vi "Secondary Master.vi"() -> ()   [LabVIEW 2021]
doc: "Secondary Modbus master that reads from a holding register periodically to ensure the primary master is functioning properly. If the holding register fails to update for a period of time, the secondary master assumes all the duties of the primary."
uses:
  Modbus_v121c/API/Modbus API.lvclass/Modbus API.ctl
  Modbus_v121c/API/Read Network Protocol.vi
  Modbus_v121c/API/Master/Modbus Master.lvclass
  D:/my_projects/projects/Algorithms/Labview/21/Modbus_v121c/API/Modbus API.lvclass
  Modbus_v121c/API/Wrapper/Create TCP Master.vi
  Stop Global.vi
  Modbus_v121c/Network Protocol/Network Master/Network Master.lvclass
  Modbus_v121c/API/Wrapper/API Main.lvlib
panel:
  out "Input Register Data":u16[](array[numeric])
  in  "Input Registers to Read":u16[](array[numeric])=[30001, 30002]
  out "Active?":bool
  in  "Heartbeat Register":u16=40001
  in  "Loop Period (ms)":u32=500
  in  "Slave Address":string="localhost"
  # "Secondary Modbus Master\n\nReads the heartbeat register that the primary master updates. If the primary master does not update the register as expected, the secondary master assumes control."
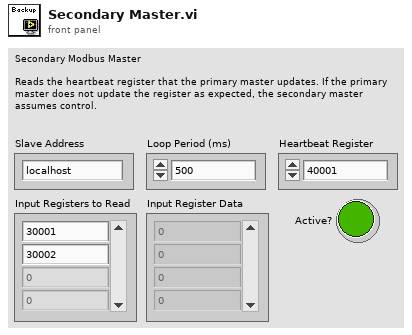
[diagram p1: front panel]
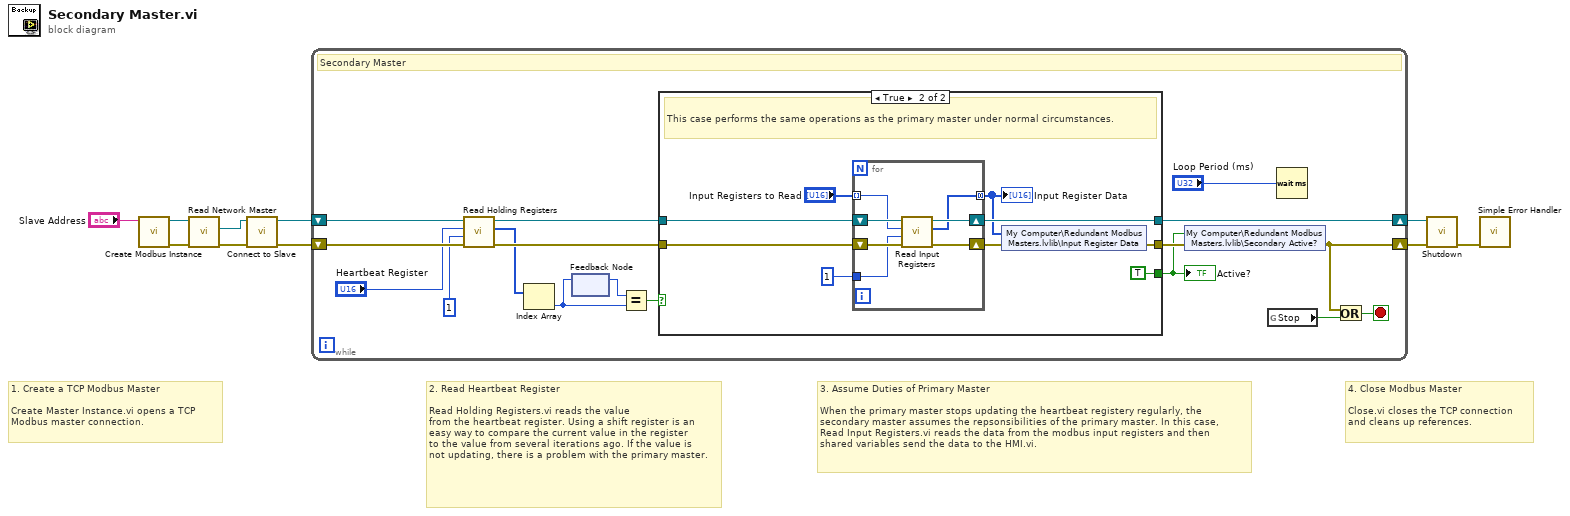
[diagram p0: block diagram]
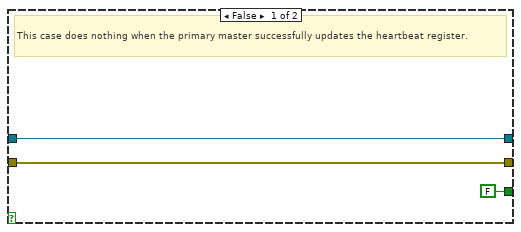
[diagram p2: hidden frame]
diagram:
  # "3. Assume Duties of Primary Master\n\nWhen the primary master stops updating the heartbeat registery regularly, the\nsecondary master assumes the repsonsibilities of the primary master. In this case,\nRead Input Registers.vi reads the data from the modbus input registers and then\nshared variables send the data to the HMI.vi."
  # "4. Close Modbus Master\n\nClose.vi closes the TCP connection\nand cleans up references."
  # "2. Read Heartbeat Register\n\nRead Holding Registers.vi reads the value\nfrom the heartbeat register. Using a shift register is an\neasy way to compare the current value in the register\nto the value from several iterations ago. If the value is\nnot updating, there is a problem with the primary master."
  # "1. Create a TCP Modbus Master\n\nCreate Master Instance.vi opens a TCP\nModbus master connection."
  n1 = call-poly "Create Modbus Instance.vi"("address"="Slave Address") -> ("error out"=w4:errorcluster, "TCP master instance"=w2:refnum<class "Modbus Master.lvclass">)  [unwired: 9 in]
  n2 = call "Read Network Master.vi"("error in"=w4, "Modbus master in"=w2) -> ("error out"=w3:errorcluster, "Network Master"=w1:refnum<class "Network Master.lvclass">)  [unwired: 7 in, 1 out]
  n3 = call-dynamic "Connect to Slave.vi"("error in (no error)"=w3, "network master in"=w1) -> ("error out"=w5:errorcluster, "network master out"=w6:refnum<class "Network Master.lvclass">)  [unwired: 8 in]
  n4 = while {
    shift-right: [w25] -> w10
    shift-left: w6 -> [w27]
    shift-right: [w22] -> w9
    shift-left: w5 -> [w26]
    stop <- w24 stop-if-true
    # "Secondary Master"
    n5 = call-dynamic "Read Holding Registers.vi"("error in (no error)"=w26, "number of holding registers"=u16 1 ("number of inputs"), "starting address"="Heartbeat Register", "Modbus master in"=w27) -> ("error out"=w20:errorcluster, "register values"=w19:u16[], "Modbus master out"=w21:refnum<class "Network Master.lvclass">)  [unwired: 5 in]
    n6 = Index Array(array=w19) -> (element=w18:u16)  [unwired: 1 in]
    n7 = feedback-in #1(w18) -> ()
    n8 = feedback #1() -> (w17:u16)  [unwired: 1 in]
    n9 = Equal?(x=w17, y=w18) -> (x = y?=w16:bool)
    n10 = case shown="True" w16 {
      tunnel: [w30 w39] -> w25
      tunnel: [w29 w38] -> w23
      tunnel: [FALSE TRUE] -> w13
      tunnel: w21 -> [w30 w37]
      tunnel: w20 -> [w29 w36]
      frame False {
        # "This case does nothing when the primary master successfully updates the heartbeat register."
      }
      frame True {
        # "This case performs the same operations as the primary master under normal circumstances."
        n11 = for {
          shift-right: [w42] -> w39
          shift-left: w37 -> [w46]
          shift-right: [w41] -> w34
          shift-left: w36 -> [w45]
          tunnel: "Input Registers to Read" -> [w44] mode=indexing
          tunnel: u16 1 -> [w43]
          tunnel: [w40] -> w31 mode=concatenating
          n12 = call-dynamic "Read Input Registers.vi"("error in (no error)"=w45, "number of input registers"=w43, "starting address"=w44, "Modbus master in"=w46) -> ("error out"=w41:errorcluster, "register values"=w40:u16[], "Modbus master out"=w42:refnum<class "Network Master.lvclass">)  [unwired: 5 in]
        }
        "Input Register Data" <- w31
        n13 = shared-variable "My Computer\\Redundant Modbus Masters.lvlib\\Input Register Data"(w31, error in=w34) -> (error out=w38:errorcluster)
      }
    }
    "Active?" <- w13
    n14 = shared-variable "My Computer\\Redundant Modbus Masters.lvlib\\Secondary Active?"(w13, error in=w23) -> (error out=w22:errorcluster)
    n15 = global read "Stop Global.vi" "Stop"() -> (w14:bool)
    n16 = Wait (ms)(milliseconds to wait="Loop Period (ms)") -> ()  [unwired: 1 out]
    n17 = Or(x=w22, y=w14) -> (x .or. y?=w24:bool)
  }
  n18 = call-dynamic "Shutdown.vi"("error in"=w9, "Network Master in"=w10) -> ("error out"=w7:errorcluster)  [unwired: 9 in]
  n19 = call <vilib>:"Simple Error Handler.vi"("error in (no error)"=w7) -> ()  [unwired: 4 in, 5 out]
